vi "Complex A x Vector (Optimized).vi"(2 "Vector":cdb[](array[numeric]) format="%.2f", 3 "A":T1) -> (0 "error":i32, 1 "A x Vector":cdb[](array[numeric]) format="%.2f")   [LabVIEW 2020, in "NI_AALBase.lvlib"]
uses:
  NI_AALBase.lvlib
  ComplexMatrix.ctl
  <resource>/lvanlys.dll
  NI_Matrix.lvlib
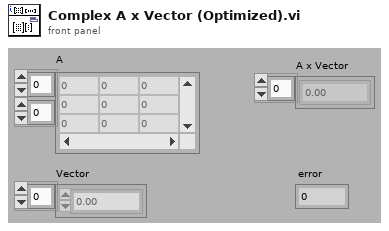
[diagram p1: front panel]
types:
  T1 = typedef "NI_Matrix.lvlib/ComplexMatrix.ctl" = cdb[][]
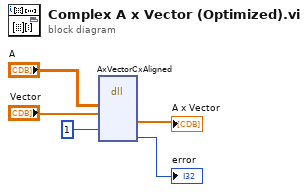
[diagram p0: block diagram]
diagram:
  n1 = dll-call lib="C:/Program Files (x86)/National Instruments/LabVIEW 2020/resource/lvanlys.*" fn="AxVectorCxAligned"("aHandle"="A", "xHandle"="Vector", "isAligned"=1) -> ("A x Vector"=→"A x Vector":cdb[], "dsperr"=→"error":i32)  [unwired: 9 in, 2 out]
